vi "2D Array to JSON.vi"(8 "error in":errorcluster, 11 "Array":dbl[][](array[numeric])) -> (0 "error out":errorcluster, 3 "String":string)   [LabVIEW 2011]
uses:
  Downloads/JSON.lvlib
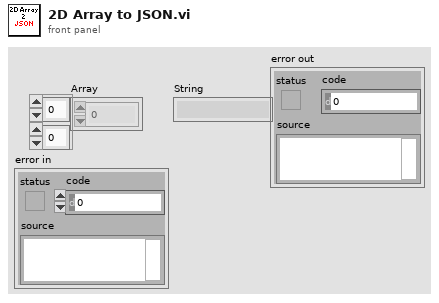
[diagram p1: front panel]
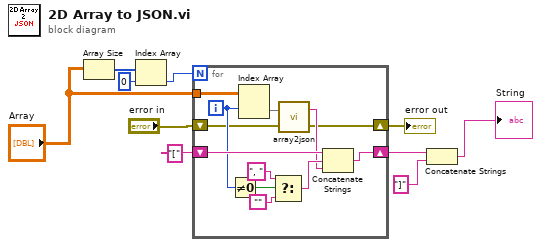
[diagram p0: block diagram]
diagram:
  n1 = Array Size(array="Array") -> (size(s)=w3:i32[])
  n2 = Index Array(array=w3, index=0) -> (element=w6:i32)
  n3 = for {
    N: w6 -> [_]
    tunnel: "Array" -> [w22]
    shift-right: [w19] -> w8
    shift-left: "[" -> [w20]
    shift-right: [w11] -> w1
    shift-left: "error in" -> [w12]
    i -> [w13]
    n4 = Not Equal To 0?(x=w13) -> (x != 0?=w17:bool)
    n5 = Index Array(array=w22, index (row)=w13) -> (element=w21:dbl[])  [unwired: 1 in]
    n6 = Select(t=", ", s=w17, f="") -> (s? t:f=w15:string)
    n7 = call "array2json.vi"("error in (no error)"=w12, "Array in"=w21) -> ("error out"=w11:errorcluster, "JSON"=w14:string)
    n8 = Concatenate Strings(w20, w15, w14) -> (w19:string)
  }
  "error out" <- w1
  n9 = Concatenate Strings(w8, "]") -> (→"String":string)
